vi "(SubVI)Scope_Receive.vi"(7 "User Code":T1 caption="Mode", 8 "error in (no error)":errorcluster caption="에러 입력(에러 없음)") -> (0 "error out":errorcluster caption="에러 출력", 2 "End":bool, 3 "Data":i16[][](array[numeric]))   [LabVIEW 2020]
uses:
  Controls/(Ctrl)Scope_Mode.ctl
  Serial/Controls/(Ctrl)Serial_Write Read Option.ctl
  Serial/Instance VIs/(SubVI)Serial_Write-Read.vi
  Serial/Instance VIs/(SubVI)Serial_Read.vi
  Serial/Controls/(Ctrl)Serial_FGV Function.ctl
panel:
  out "ff?":bool
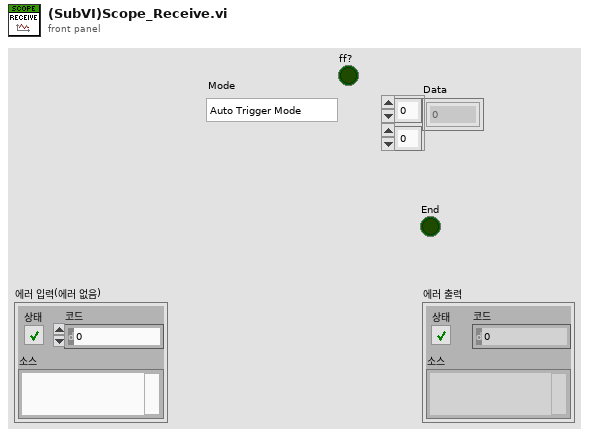
[diagram p1: front panel]
types:
  T1 = typedef "(Ctrl)Scope_Mode.ctl" = enum8{"Auto Trigger Mode", "Continuous Mode"}
  T2 = typedef "(Ctrl)Serial_FGV Function.ctl" = enum16{"Initialize", "Read", "Read All", "Write", "Flush Buffer", "Get Ref.", "Close"}
  T3 = typedef "(Ctrl)Serial_Write Read Option.ctl" = cluster{"Echo Request":bool, "Header Verification":bool, "Checksum Verification":bool, "User Code Verifiaction":bool}
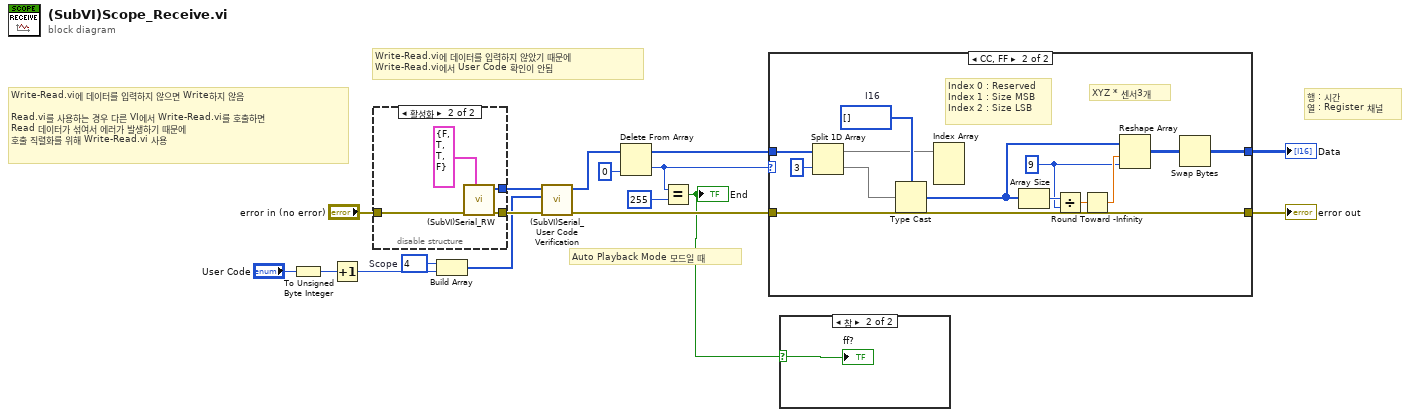
[diagram p0: block diagram]
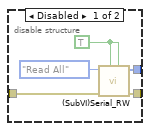
[diagram p3: hidden frame]
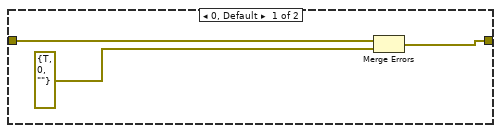
[diagram p4: hidden frame]
diagram:
  w15 = u8 4  # Scope
  # "Auto Playback Mode 모드일 때"
  # "Write-Read.vi에 데이터를 입력하지 않았기 때문에\nWrite-Read.vi에서 User Code 확인이 안됨"
  # "Write-Read.vi에 데이터를 입력하지 않으면 Write하지 않음\n\nRead.vi를 사용하는 경우 다른 VI에서 Write-Read.vi를 호출하면\nRead 데이터가 섞여서 에러가 발생하기 때문에\n호출 직렬화를 위해 Write-Read.vi 사용"
  # "행 : 시간\n열 : Register 채널"
  n1 = To Unsigned Byte Integer(number="User Code") -> (unsigned 8bit integer=w5:u8)
  n2 = Increment(x=w5) -> (x+1=w4:u8)
  n3 = disable-structure shown="활성화" {
    disable-tunnel: "error in (no error)" -> [w22 w26]
    disable-tunnel: [w21 w25] -> w14
    disable-tunnel: [w20 w24] -> w8
    frame Disabled {
      w19 = TRUE ("Header Verification")
      n4 = call-poly "(SubVI)Serial_RW.vi"("Checksum Verification"=w19, "Header Verification"=w19, "error in (no error)"=w22, "Function"=(Ctrl)Serial_FGV_Function."Read All") -> ("error out"=w21:errorcluster, "Read Data"=w20:u8[])  [unwired: 5 in, 1 out]
    }
    frame Enabled {
      n5 = call-poly "(SubVI)Serial_RW.vi"("Option"=T3 {"Echo Request"=FALSE, "Header Verification"=TRUE, "Checksum Verification"=TRUE, "User Code Verifiaction"=FALSE}, "error in (no error)"=w26) -> ("error out"=w25:errorcluster, "Read Data"=w24:u8[])  [unwired: 7 in, 1 out]
    }
  }
  n6 = Build Array(w15, w4) -> (w7:u8[])
  n7 = call "(SubVI)Serial_User Code Verification.vi"("에러 입력(에러 없음)"=w14, "Data to Write"=w7, "Read Data"=w8) -> ("에러 출력"=w9:errorcluster, "Read Data"=w6:u8[])  [unwired: 7 in]
  n8 = Delete From Array(array=w6, index=0 ("인덱스")) -> (deleted portion=w3:u8, array with subset deleted=w11:u8[])  [unwired: 1 in]
  n9 = Equal?(x=w3, y=u8 255) -> (x = y?=w1:bool)
  "End" <- w1
  n10 = case shown="CC, FF" w3 {
    tunnel: w9 -> [w29 w42]
    tunnel: [w28 w42] -> w12
    tunnel: w11 -> [_ w35]
    tunnel: [_ w30] -> w10
    frame 0, Default {
      n11 = Merge Errors(w29, errorcluster {"status"=TRUE, "code"=0, "source"=""} ("에러 입력")) -> (w28:errorcluster)
    }
    frame 204, 255 {
      w31 = 9 ("차원 크기")
      w40 = i16[] []  # I16
      # "XYZ * 센서3개"
      # "Index 0 : Reserved\nIndex 1 : Size MSB\nIndex 2 : Size LSB"
      n12 = Split 1D Array(array=w35, index=3 ("인덱스")) -> (first subarray=w32:u8[], second subarray=w34:u8[])
      n13 = Type Cast(type=w40, x=w34) -> (*(type *) &x=w33:i16[])
      n14 = Index Array(array=w32) -> ()  [unwired: 3 in, 3 out]
      n15 = Array Size(array=w33) -> (size(s)=w36:i32)
      n16 = Divide(x=w36, y=w31) -> (x/y=w37:dbl)
      n17 = Round Toward -Infinity(1:w37) -> (0:w38:dbl)
      n18 = Reshape Array(w33, w38, w31) -> (w41:i16[][])
      n19 = Swap Bytes(anything=w41) -> (byte swapped=w30:i16[][])
    }
  }
  "error out" <- w12
  "Data" <- w10
  n20 = case shown="참" w1 {
    selector: w1 -> [_ w43]
    frame False {
    }
    frame True {
      "ff?" <- w43
    }
  }
